vi "joypad.vi"() -> ()   [LabVIEW 2021]
uses:
  <vilib>/Utility/inputDevices.llb/joystickAcquire.vi
  <vilib>/Utility/inputDevices.llb/closeJoystick.vi
panel:
  out "Angle":dbl
  out "Magnitude":dbl
  out "coerced(x) 2":dbl
  out "coerced(x)":dbl
  out "x+y 2":dbl
  out "x+y":dbl
  out "direction info":T1
  out "button info":T2
  out "axis info":T3
  in  "stop":bool
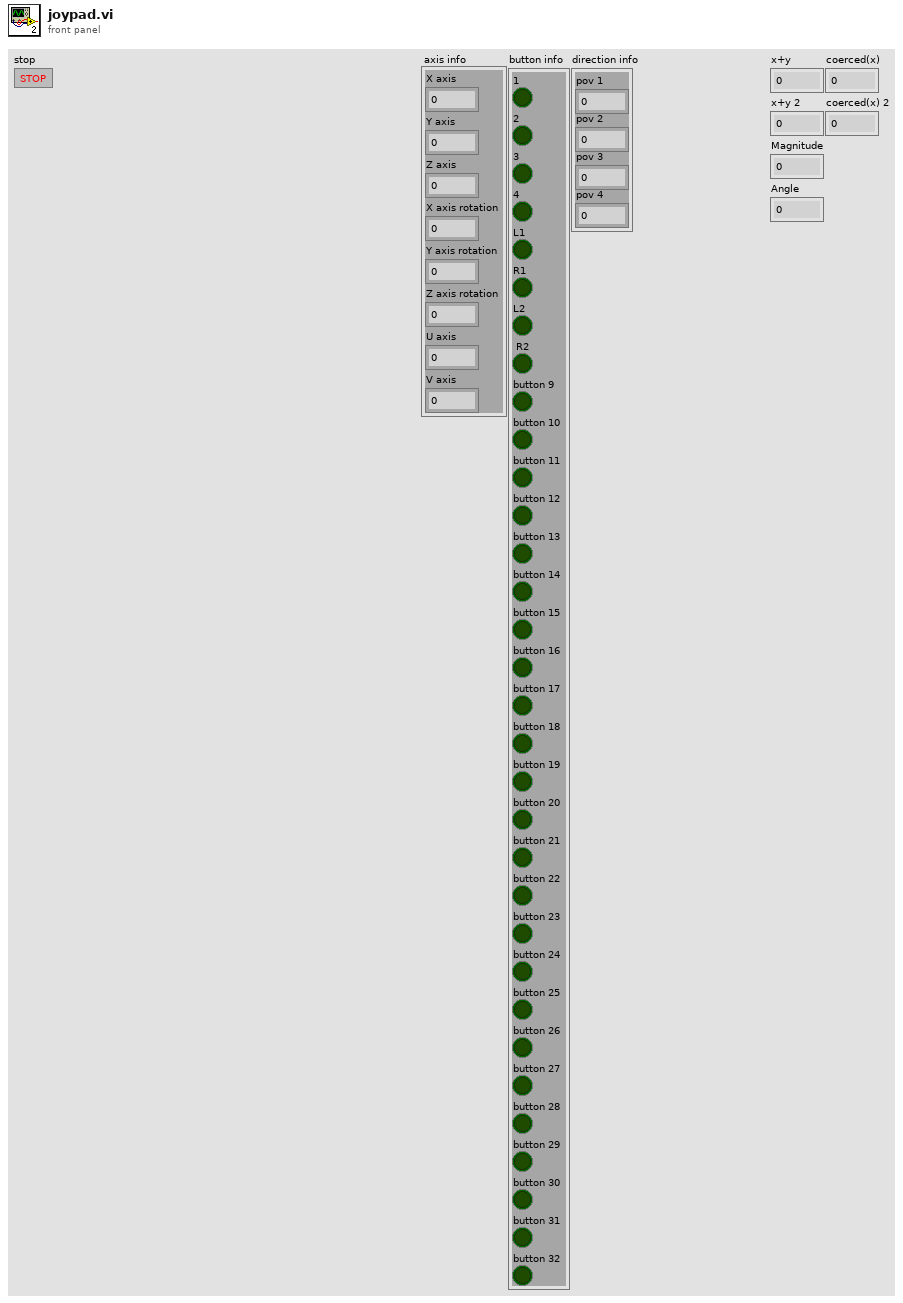
[diagram p1: front panel]
types:
  T1 = cluster{"pov 1":i32, "pov 2":i32, "pov 3":i32, "pov 4":i32}
  T2 = cluster{"1":bool, "2":bool, "3":bool, "4":bool, "L1":bool, "R1":bool, "L2":bool, " R2":bool, "button 9":bool, "button 10":bool, "button 11":bool, "button 12":bool, "button 13":bool, "button 14":bool, "button 15":bool, "button 16":bool, "button 17":bool, "button 18":bool, "button 19":bool, "button 20":bool, "button 21":bool, "button 22":bool, "button 23":bool, "button 24":bool, "button 25":bool, "button 26":bool, "button 27":bool, "button 28":bool, "button 29":bool, "button 30":bool, "button 31":bool, "button 32":bool}
  T3 = cluster{"X axis":i32, "Y axis":i32, "Z axis":i32, "X axis rotation":i32, "Y axis rotation":i32, "Z axis rotation":i32, "U axis":i32, "V axis":i32}
  T4 = cluster{"button 1":bool, "button 2":bool, "button 3":bool, "button 4":bool, "button 5":bool, "button 6":bool, "button 7":bool, "button 8":bool, "button 9":bool, "button 10":bool, "button 11":bool, "button 12":bool, "button 13":bool, "button 14":bool, "button 15":bool, "button 16":bool, "button 17":bool, "button 18":bool, "button 19":bool, "button 20":bool, "button 21":bool, "button 22":bool, "button 23":bool, "button 24":bool, "button 25":bool, "button 26":bool, "button 27":bool, "button 28":bool, "button 29":bool, "button 30":bool, "button 31":bool, "button 32":bool}
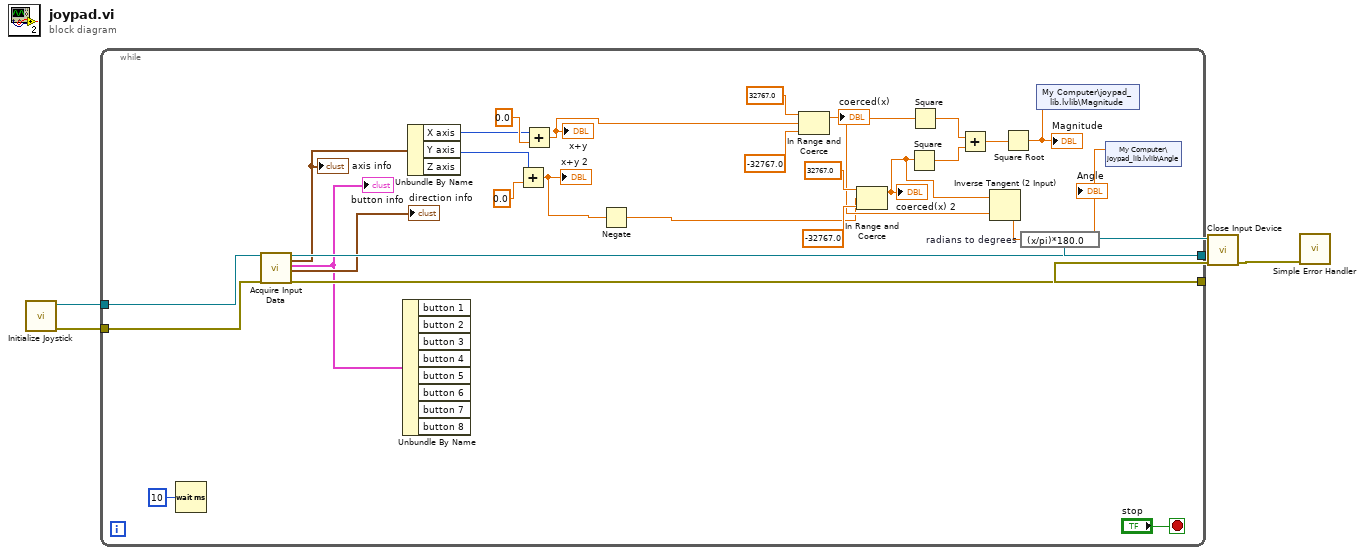
[diagram p0: block diagram]
diagram:
  n1 = call <vilib>:"Initialize Joystick.vi"() -> ("error out"=w4:errorcluster, "device ID"=w5:refnum<k1>)  [unwired: 10 in]
  n2 = while {
    tunnel: w5 -> [w32]
    tunnel: w4 -> [w31]
    tunnel: [w30] -> w3
    tunnel: [w29] -> w2
    stop <- "stop" stop-if-true
    n3 = Wait (ms)(milliseconds to wait=u32 10) -> ()  [unwired: 1 out]
    n4 = call-poly <vilib>:"Acquire Input Data.vi"("device ID"=w32, "error in (no error)"=w31) -> ("device ID"=w30:refnum<k1>, "axis info"=w27:T3, "button info"=w6:T4, "direction info"=→"direction info":T1, "error out"=w29:errorcluster)  [unwired: 13 in]
    "axis info" <- w27
    "button info" <- w6
    n5 = Unbundle By Name(w6) -> ()  [unwired: 8 out]
    n6 = Unbundle By Name(w27) -> ("X axis"=w20:i32, "Y axis"=w24:i32)  [unwired: 1 out]
    n7 = Add(x=w24, y=0.0) -> (x+y=w7:dbl)
    "x+y 2" <- w7
    n8 = Add(x=w20, y=0.0) -> (x+y=w23:dbl)
    "x+y" <- w23
    n9 = Negate(x=w7) -> (-x=w8:dbl)
    n10 = In Range and Coerce(upper limit=32767.0, x=w23, lower limit=-32767.0) -> (coerced(x)=w12:dbl)  [unwired: 1 out]
    "coerced(x)" <- w12
    n11 = In Range and Coerce(upper limit=32767.0, x=w8, lower limit=-32767.0) -> (coerced(x)=w13:dbl)  [unwired: 1 out]
    "coerced(x) 2" <- w13
    n12 = Square(x=w13) -> (x^2=w17:dbl)
    n13 = Square(x=w12) -> (x^2=w16:dbl)
    n14 = Add(x=w16, y=w17) -> (x+y=w15:dbl)
    n15 = Inverse Tangent (2 Input)(1:w12, 2:w13) -> (0:w11:dbl)
    n16 = Square Root(x=w15) -> (sqrt(x)=w14:dbl)
    "Magnitude" <- w14
    n17 = expression code="(x/pi)*180.0" "radians to degrees"(w11) -> (w10:dbl)
    "Angle" <- w10
    n18 = shared-variable "My Computer\\joypad_lib.lvlib\\Magnitude"(w14) -> ()  [unwired: 1 in, 1 out]
    n19 = shared-variable "My Computer\\joypad_lib.lvlib\\Angle"(w10) -> ()  [unwired: 1 in, 1 out]
  }
  n20 = call-poly <vilib>:"Close Input Device.vi"("error in (no error)"=w2, "device ID"=w3) -> ("error out"=w1:errorcluster)  [unwired: 8 in]
  n21 = call <vilib>:"Simple Error Handler.vi"("error in (no error)"=w1) -> ()  [unwired: 4 in, 5 out]
